vi "channel.get.vi"(8 "error in":errorcluster, 9 "name":string, 10 "data source rid":string, 11 "Client in":refnum<class "Client.lvclass">) -> (0 "error out":errorcluster, 2 "Channel":refnum<class "Channel.lvclass">, 3 "Client out":refnum<class "Client.lvclass">)   [LabVIEW 2020, in "Client.lvclass"]
doc: "Fetches a specific channel's metadata by data source and channel name."
uses:
  Client.lvclass
  Client.lvclass/Client.ctl
  client.lvlib
  Channel/Channel.lvclass
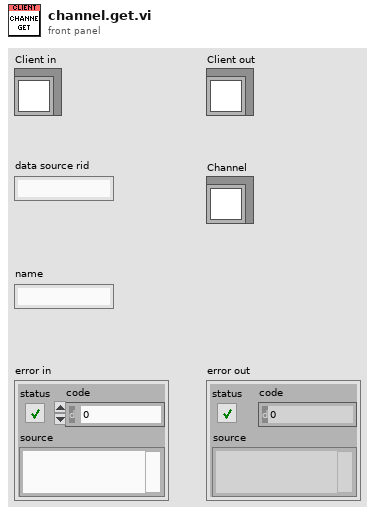
[diagram p1: front panel]
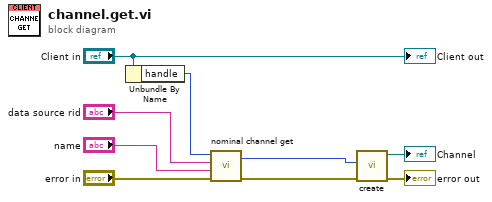
[diagram p0: block diagram]
diagram:
  n1 = Unbundle By Name("Client in") -> ("handle"=w8:i32)
  n2 = call "nominal channel get.vi"("error in (no error)"="error in", "name"="name", "data_source_rid"="data source rid", "client"=w8) -> ("error out"=w3:errorcluster, "out_channel out"=w4:i32)  [unwired: 5 in, 1 out]
  n3 = call "create.vi"("error in (no error)"=w3, "handle"=w4) -> ("error out"=→"error out":errorcluster, "Channel"=→"Channel":refnum<class "Channel.lvclass">)  [unwired: 8 in]
  "Client out" <- "Client in"
